vi "Get Class Column Ordering - Full.vi"(8 "error in (no error)":errorcluster {"code" format="Error %.0f"}, 11 "VIDoc Printer - Confluence In":refnum<class "VIDoc Printer - Confluence.lvclass">) -> (0 "error out":errorcluster {"code" format="Error %.0f"}, 2 "Full":T1[](array[typedef]), 3 "VIDoc Printer - Confluence Out":refnum<class "VIDoc Printer - Confluence.lvclass">)   [LabVIEW 2023, in "VIDoc Printer - Confluence.lvlib" / "VIDoc Printer - Confluence.lvclass"]
uses:
  VIDoc Printer - Confluence.lvclass
  Settings/Confluence Printer Settings/Class Info Column.ctl
  VIDoc Printer - Confluence.lvclass/VIDoc Printer - Confluence.ctl
  Settings/Confluence Printer Settings/VIDoc Settings - Confluence.lvclass
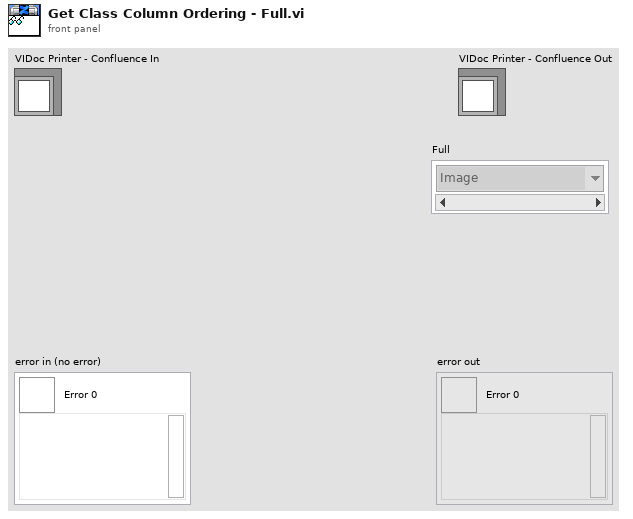
[diagram p1: front panel]
types:
  T1 = typedef "VIDoc Printer - Confluence.lvlib/VIDoc Settings - Confluence.lvclass/Class Info Column.ctl" = enum16{"Image", "Name", "Description", "Version", "Last Change", "Author", "Commit Hash", "Branch", "Qualified Name", "TransferMustOverrides", "ChildRefsRestricted"}
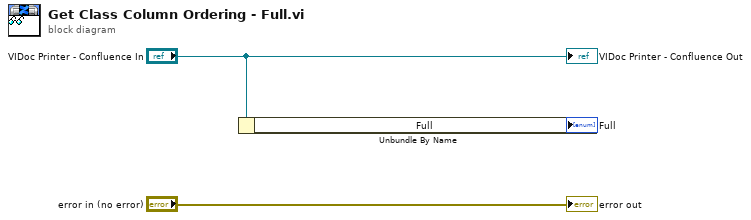
[diagram p0: block diagram]
diagram:
  n1 = Unbundle By Name("VIDoc Printer - Confluence In") -> ("Full"=→"Full":T1[])
  "error out" <- "error in (no error)"
  "VIDoc Printer - Confluence Out" <- "VIDoc Printer - Confluence In"
